vi "Configuration SubVI.vi"(8 "error in (no error)":errorcluster, 11 "Simulation in":refnum<class "Simulation.lvclass">) -> (0 "error out":errorcluster, 3 "Simulation out":refnum<class "Simulation.lvclass">)   [LabVIEW 2020, in "I2C Storage.lvlib" / "Simulation.lvclass"]
uses:
  Simulation.lvclass
  Parent/I2C Storage.lvclass
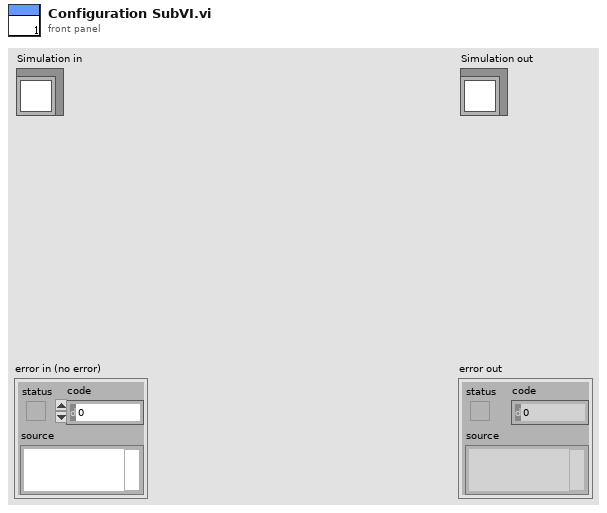
[diagram p1: front panel]
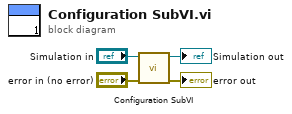
[diagram p0: block diagram]
diagram:
  n1 = call-parent "Configuration SubVI.vi"("error in (no error)"="error in (no error)", "Devices in"="Simulation in") -> ("error out"=→"error out":errorcluster, "Devices out"=→"Simulation out":refnum<class "Simulation.lvclass">)  [unwired: 8 in]
